vi "Rohde & Schwarz VNA Compute Timeout.vi"(5 "Points":i32, 7 "IFBW (Hz)":dbl, 9 "Sweep Time (s)":dbl) -> (8 "Timeout (ms)":u32)   [LabVIEW 2011]
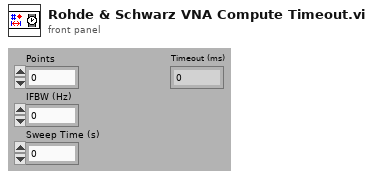
[diagram p1: front panel]
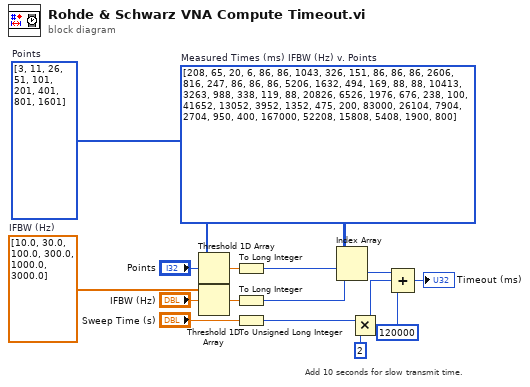
[diagram p0: block diagram]
diagram:
  w8 = dbl[] [10.0, 30.0, 100.0, 300.0, 1000.0, 3000.0]  # IFBW (Hz)
  w9 = i32[] [3, 11, 26, 51, 101, 201, 401, 801, 1601]  # Points
  w16 = u32[][] [[208, 65, 20, 6, 86, 86], [1043, 326, 151, 86, 86, 86], [2606, 816, 247, 86, 86, 86], [5206, 1632, 494, 169, 88, 88], [10413, 3263, 988, 338, 119, 88], [20826, 6526, 1976, 676, 238, 100], [41652, 13052, 3952, 1352, 475, 200], [83000, 26104, 7904, 2704, 950, 400], [167000, 52208, 15808, 5408, 1900, 800]]  # Measured Times (ms) IFBW (Hz) v. Points
  # "Add 10 seconds for slow transmit time."
  n1 = Threshold 1D Array(2:"Points", 3:w9) -> (0:w15:dbl)  [unwired: 1 out]
  n2 = Threshold 1D Array(2:"IFBW (Hz)", 3:w8) -> (0:w12:dbl)  [unwired: 1 out]
  n3 = To Long Integer(number=w15) -> (32bit integer=w13:i32)
  n4 = To Long Integer(number=w12) -> (32bit integer=w11:i32)
  n5 = To Unsigned Long Integer(number="Sweep Time (s)") -> (unsigned 32bit integer=w2:u32)
  n6 = Index Array(array=w16, index (row)=w13, index (col)=w11) -> (element=w6:u32)
  n7 = Multiply(x=w2, y=2) -> (x*y=w1:u32)
  n8 = Compound Arithmetic op=ADD(w6, w1, u32 120000 ("y")) -> (→"Timeout (ms)":u32)
